vi "Render Escaped Tag-Text.vi"(8 "Error In":errorcluster) -> (0 "Error Out":errorcluster)   [LabVIEW 2018, in "Tests.lvlib" / "Render.lvlib"]
uses:
  Render.lvlib
  src/Toolkit/Data/Map/Map.lvclass
  D:/Users/cfield/Code/Field R&D Services/Mustache/LabVIEW/trunk/src/Toolkit/Data/Abstract/Abstract.lvclass
  src/Toolkit/Low-Level/Support/Lex String.vi
  src/Toolkit/Data/Map/Support/From String.vi
  src/Toolkit/Low-Level/Support/Render to String.vi
  <vilib>/addons/_JKI Toolkits/Caraya/classes/Test/Test.lvclass
  <vilib>/addons/_JKI Toolkits/Caraya/classes/Assert/Assert.lvclass
  src/Toolkit/Toolkit.lvlib
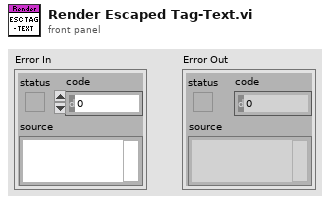
[diagram p1: front panel]
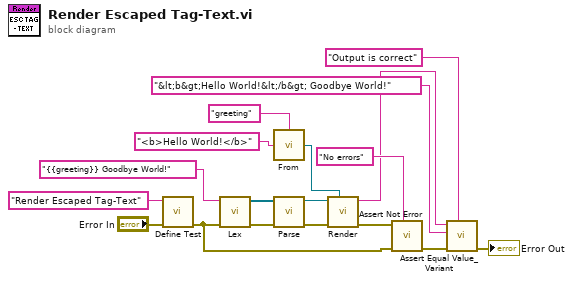
[diagram p0: block diagram]
diagram:
  n1 = call <vilib>:"Define Test.vi"("error in (no error)"="Error In", "Label (VI Title)"="Render Escaped Tag-Text") -> ("error out"=w2:errorcluster)  [unwired: 9 in]
  n2 = call-poly "Lex.vi"("Error In"=w2, "Input"="{{greeting}} Goodbye World!" ("format string")) -> ("Error Out"=w11:errorcluster, "Tokens"=w10:refnum<class "Abstract.lvclass">[])  [unwired: 8 in]
  n3 = call-poly "From.vi"("Value"="<b>Hello World!</b>", "Key"="greeting") -> ("Map"=w5:refnum<class "Map.lvclass">)
  n4 = call "Parse.vi"("Error In"=w11, "Tokens"=w10) -> ("Error Out"=w9:errorcluster, "Abstract Syntax Tree"=w8:refnum<class "Root.lvclass">)  [unwired: 8 in]
  n5 = call-poly "Render.vi"("Data"=w5, "Error In"=w9, "Abstract Syntax Tree"=w8) -> ("Error Out"=w7:errorcluster, "Output"=w6:string)  [unwired: 7 in]
  n6 = call <vilib>:"Assert Not Error.vi"("Label"="No errors", "error in (no error)"=w2, "Not Error?"=w7) -> ("error out"=w15:errorcluster)  [unwired: 8 in]
  n7 = call <vilib>:"Assert Equal Value_Variant.vi"("Label"="Output is correct", "error in (no error)"=w15, "Y"="&lt;b&gt;Hello World!&lt;/b&gt; Goodbye World!" ("Value"), "X"=w6) -> ("error out"=→"Error Out":errorcluster)  [unwired: 7 in]
